vi "Initialize Interface Sessions.vi"(8 "error in (no error)":errorcluster, 11 "PXImc Transceiver in":refnum<class "DSF PXImc Transceiver.lvclass">=refnum) -> (0 "error out":errorcluster, 3 "PXImc Transceiver out":refnum<class "DSF PXImc Transceiver.lvclass">)   [LabVIEW 2017, in "DSF Core.lvlib" / "DSF PXImc Transceiver.lvclass"]
uses:
  DSF PXImc Transceiver.lvclass
  DSF PXImc Transceiver.lvclass/DSF PXImc Transceiver.ctl
  <vilib>/pximc/Initialize Writer Session (U8).vi
  <vilib>/pximc/Initialize Reader Session (U8).vi
  <vilib>/pximc/nipximc.lvlib
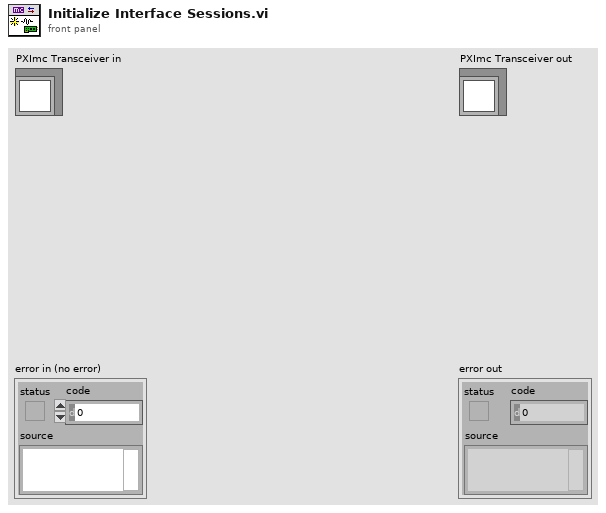
[diagram p1: front panel]
types:
  T1 = typedef "DSF Core.lvlib/DSF PXImc Transceiver.lvclass/PXImc Group Data.ctl" = cluster{"direction":T2, "transfers":T3[]}
  T2 = typedef "DSF Core.lvlib/DSF Direction.ctl" = enum8{"Tx", "Rx"}
  T3 = typedef "DSF Core.lvlib/DSF PXImc Transceiver.lvclass/PXImc Transfer Data.ctl" = cluster{"stream id":u16, "session":refnum<k21>, "buffer size":u64}
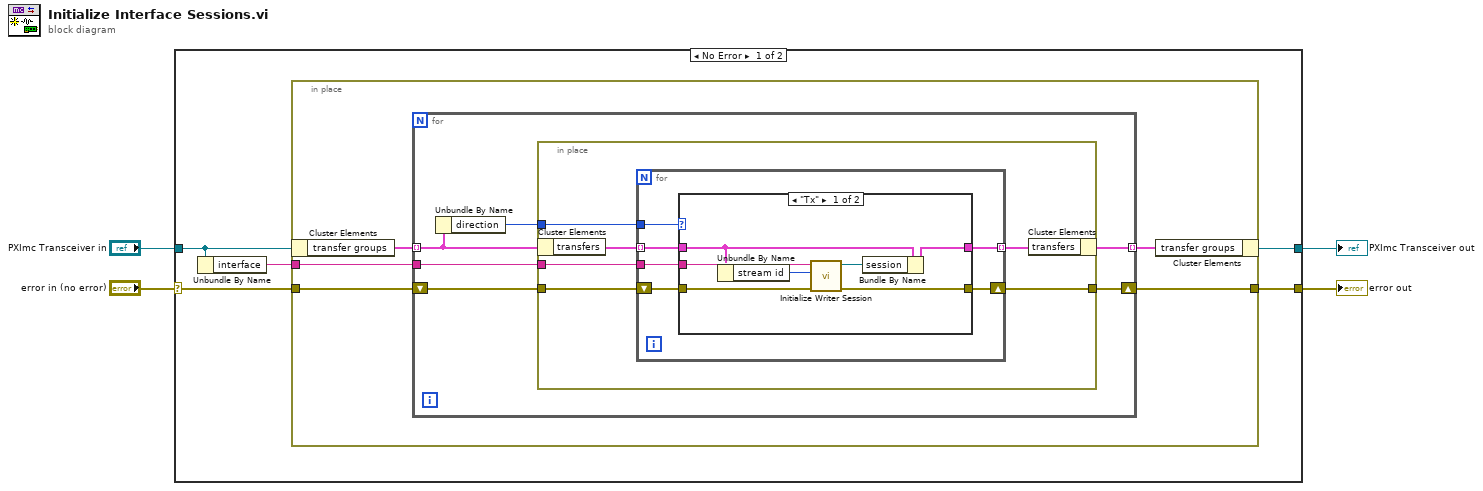
[diagram p0: block diagram]
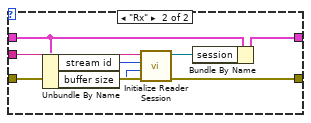
[diagram p2: hidden frame]
diagram:
  n1 = case shown="No Error" "error in (no error)" {
    selector: "error in (no error)" -> [w9 w49]
    tunnel: [w7 w49] -> w3
    tunnel: [w5 w48] -> w1
    tunnel: "PXImc Transceiver in" -> [w6 w48]
    frame No Error {
      n2 = Unbundle By Name(w6) -> ("interface"=w8:tag)
      n3 = in-place {
        in-place-border: w9 -> [w14]
        in-place-border: w8 -> [w13]
        in-place-border: [w12] -> w7
        n4 = in-place-cluster #1(w6) -> ("transfer groups"=w11:T1[])
        n5 = for {
          tunnel: w11 -> [w16] mode=indexing
          shift-right: [w19] -> w12
          shift-left: w14 -> [w20]
          tunnel: w13 -> [w18]
          tunnel: [w17] -> w10 mode=indexing
          n6 = Unbundle By Name(w16) -> ("direction"=w15:T2)
          n7 = in-place {
            in-place-border: w20 -> [w26]
            in-place-border: [w25] -> w19
            in-place-border: w18 -> [w24]
            in-place-border: w15 -> [w21]
            n8 = in-place-cluster #2(w16) -> ("transfers"=w23:T3[])
            n9 = for {
              tunnel: w24 -> [w30]
              tunnel: w23 -> [w29] mode=indexing
              shift-right: [w31] -> w25
              shift-left: w26 -> [w32]
              tunnel: [w28] -> w22 mode=indexing
              tunnel: w21 -> [w27]
              n10 = case shown="\"Tx\"" w27 {
                tunnel: w32 -> [w39 w47]
                tunnel: [w38 w46] -> w31
                tunnel: w30 -> [w37 w45]
                tunnel: w29 -> [w35 w43]
                tunnel: [w34 w42] -> w28
                frame "Tx" {
                  n11 = Unbundle By Name(w35) -> ("stream id"=w33:u16)
                  n12 = call-poly <vilib>:"Initialize Writer Session.vi"("error in (no error)"=w39, "connection id (1)"=w33, "interface"=w37) -> ("error out"=w38:errorcluster, "session out"=w36:refnum<k21>)  [unwired: 7 in]
                  n13 = Bundle By Name(cluster=w35, "session"=w36) -> (w34:T3)
                }
                frame "Rx" {
                  n14 = Unbundle By Name(w43) -> ("stream id"=w41:u16, "buffer size"=w40:u64)
                  n15 = call-poly <vilib>:"Initialize Reader Session.vi"("error in (no error)"=w47, "buffer size"=w40, "writer's connection id (1)"=w41, "interface"=w45) -> ("error out"=w46:errorcluster, "session out"=w44:refnum<k21>)  [unwired: 6 in]
                  n16 = Bundle By Name(cluster=w43, "session"=w44) -> (w42:T3)
                }
              }
            }
            n17 = in-place-cluster #2("transfers"=w22) -> (w17:T1)
          }
        }
        n18 = in-place-cluster #1("transfer groups"=w10) -> (w5:refnum<class "DSF PXImc Transceiver.lvclass">)
      }
    }
    frame Error {
    }
  }
  "error out" <- w3
  "PXImc Transceiver out" <- w1
